vi "Create Channels.vi"(8 "error in (no error)":errorcluster) -> (0 "error out":errorcluster, 3 "Device Item Ref out":T3 format="%.0x")   [LabVIEW 2011, in "IVI DC Power Supply Custom Device.lvlib"]
uses:
  IVI DC Power Supply Custom Device.lvlib
  <vilib>/NI Veristand/Custom Device API/Custom Device Item Ref.ctl
  <vilib>/NI Veristand/Custom Device API/Custom Device Channel.ctl
  <vilib>/NI Veristand/Custom Device API/Custom Device Channel Type.ctl
  current behaviour.ctl
  Global.vi
  <vilib>/NI Veristand/Custom Device Tools/Custom Device Utility Library/NI VeriStand - Search for All Items by GUID.vi
  <vilib>/NI Veristand/Custom Device API/Set Item Property (U16).vi
  <vilib>/NI Veristand/Custom Device API/Get Item Property (U16).vi
  <vilib>/NI Veristand/Custom Device API/Custom Device API.lvlib
  <vilib>/NI Veristand/Custom Device Tools/Custom Device Utility Library/Custom Device Utility Library.lvlib
panel:
  in  "Output Channel":T1={"Type"=enum."Output", "Units"="", "Default Value"=0.0, "Faultable"=FALSE, "Scalable"=FALSE}
  in  "Input Channel":T1
  in  "Node Ptr":T3 format="%.0x"
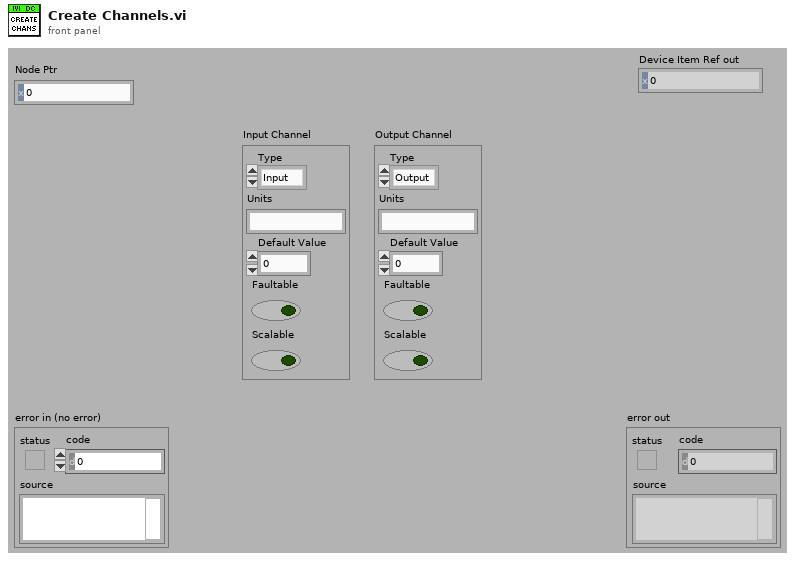
[diagram p1: front panel]
types:
  T1 = typedef "Custom Device API.lvlib/Custom Device Channel.ctl" = cluster{"Type":T2, "Units":string, "Default Value":dbl, "Faultable":bool, "Scalable":bool}
  T2 = typedef "Custom Device API.lvlib/Custom Device Channel Type.ctl" = enum16{"Input", "Output"}
  T3 = typedef "Custom Device API.lvlib/Custom Device Item Ref.ctl" = u64
  T4 = typedef "IVI DC Power Supply Custom Device.lvlib/current behaviour.ctl" = enum16{"Regulate", "Trip"}
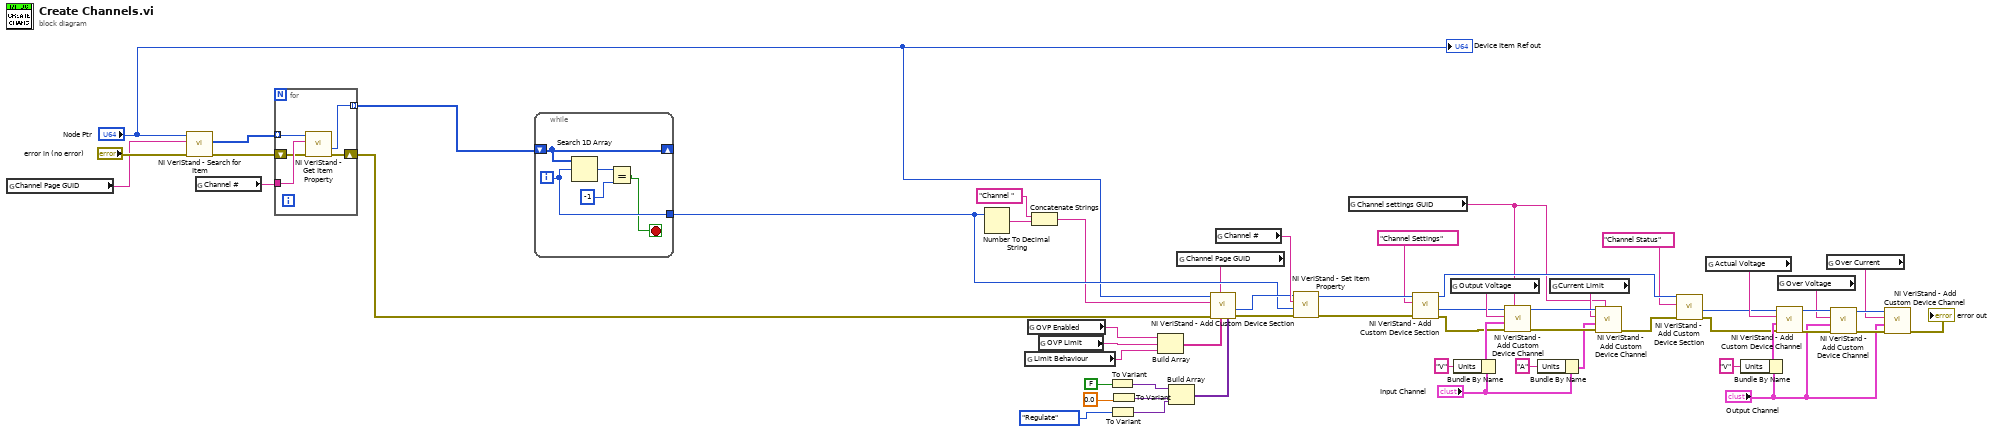
[diagram p0: block diagram]
diagram:
  n1 = global read "Global.vi" "Channel Page GUID"() -> (w1:string)
  n2 = call-poly <vilib>:"NI VeriStand - Search for Item.vi"("error in"="error in (no error)", "Item GUID"=w1, "Section Ref in"="Node Ptr") -> ("error out"=w2:errorcluster, "Item Refs"=w5:T3[])  [unwired: 5 in, 2 out]
  n3 = global read "Global.vi" "Channel #"() -> (w57:string)
  n4 = for {
    tunnel: w57 -> [w63]
    tunnel: w5 -> [w62] mode=indexing
    shift-right: [w60] -> w58
    shift-left: w2 -> [w61]
    tunnel: [w59] -> w6 mode=indexing
    n5 = call-poly <vilib>:"NI VeriStand - Get Item Property.vi"("error in (no error)"=w61, "Property Name"=w63, "Item Ref in"=w62) -> ("error out"=w60:errorcluster, "Value"=w59:u16)  [unwired: 5 in, 2 out]
  }
  n6 = while {
    shift-right: [w66] -> _
    shift-left: w6 -> [w66]
    tunnel: [w65] -> w46
    i -> [w65]
    stop <- w64 stop-if-true
    n7 = Search 1D Array(1D array=w66, element=w65) -> (index of element=w68:i32)  [unwired: 1 in]
    n8 = Equal?(x=w68, y=-1) -> (x = y?=w64:bool)
  }
  n9 = Number To Decimal String(number=w46) -> (decimal integer string=w49:string)  [unwired: 1 in]
  n10 = global read "Global.vi" "Limit Behaviour"() -> (w11:string)
  n11 = global read "Global.vi" "OVP Enabled"() -> (w56:string)
  n12 = Concatenate Strings("Channel " ("string"), w49) -> (w45:string)
  n13 = global read "Global.vi" "OVP Limit"() -> (w53:string)
  n14 = To Variant(anything=FALSE) -> (Variant=w55:variant)
  n15 = To Variant(anything=current_behaviour."Regulate" ("Enum")) -> (Variant=w9:variant)
  n16 = To Variant(anything=0.0) -> (Variant=w52:variant)
  n17 = Build Array(w56, w53, w11) -> (w39:string[])
  n18 = Build Array(w55, w52, w9) -> (w38:variant[])
  n19 = global read "Global.vi" "Channel Page GUID"() -> (w44:string)
  n20 = call <vilib>:"NI VeriStand - Add Custom Device Section.vi"("Property Values"=w38, "Property names"=w39, "GUID (Default Section)"=w44, "error in (no error)"=w58, "Section Name"=w45, "Parent Ref in"="Node Ptr") -> ("error out"=w51:errorcluster, "Section Ptr"=w47:T3)  [unwired: 2 in, 2 out]
  n21 = global read "Global.vi" "Channel #"() -> (w50:string)
  n22 = call-poly <vilib>:"NI VeriStand - Set Item Property.vi"("error in (no error)"=w51, "Value"=w46, "Property Name"=w50, "Item Ref in"=w47) -> ("error out"=w21:errorcluster, "Item Ref out"=w18:T3)  [unwired: 5 in, 1 out]
  n23 = global read "Global.vi" "Channel settings GUID"() -> (w7:string)
  n24 = call <vilib>:"NI VeriStand - Add Custom Device Section.vi"("error in (no error)"=w21, "Section Name"="Channel Settings", "Parent Ref in"=w18) -> ("error out"=w20:errorcluster, "Section Ptr"=w19:T3, "Parent Ref out"=w13:T3)  [unwired: 5 in, 1 out]
  n25 = global read "Global.vi" "Output Voltage"() -> (w42:string)
  n26 = Bundle By Name(cluster="Input Channel", "Units"="V") -> (w28:T1)
  n27 = call <vilib>:"NI VeriStand - Add Custom Device Channel.vi"("GUID (Default Channel)"=w7, "error in (no error)"=w20, "Channel"=w28, "Channel Name"=w42, "Parent Ref in"=w19) -> ("error out"=w40:errorcluster, "Parent Ref out"=w43:T3)  [unwired: 3 in, 2 out]
  n28 = Bundle By Name(cluster="Input Channel", "Units"="A") -> (w27:T1)
  n29 = global read "Global.vi" "Current Limit"() -> (w41:string)
  n30 = call <vilib>:"NI VeriStand - Add Custom Device Channel.vi"("GUID (Default Channel)"=w7, "error in (no error)"=w40, "Channel"=w27, "Channel Name"=w41, "Parent Ref in"=w43) -> ("error out"=w16:errorcluster)  [unwired: 3 in, 3 out]
  n31 = call <vilib>:"NI VeriStand - Add Custom Device Section.vi"("error in (no error)"=w16, "Section Name"="Channel Status", "Parent Ref in"=w13) -> ("error out"=w15:errorcluster, "Section Ptr"=w14:T3)  [unwired: 5 in, 2 out]
  n32 = global read "Global.vi" "Actual Voltage"() -> (w32:string)
  n33 = Bundle By Name(cluster="Output Channel", "Units"="V") -> (w22:T1)
  n34 = call <vilib>:"NI VeriStand - Add Custom Device Channel.vi"("error in (no error)"=w15, "Channel"=w22, "Channel Name"=w32, "Parent Ref in"=w14) -> ("error out"=w35:errorcluster, "Parent Ref out"=w34:T3)  [unwired: 4 in, 2 out]
  n35 = global read "Global.vi" "Over Voltage"() -> (w31:string)
  n36 = global read "Global.vi" "Over Current"() -> (w30:string)
  n37 = call <vilib>:"NI VeriStand - Add Custom Device Channel.vi"("error in (no error)"=w35, "Channel"="Output Channel", "Channel Name"=w31, "Parent Ref in"=w34) -> ("error out"=w36:errorcluster, "Parent Ref out"=w33:T3)  [unwired: 4 in, 2 out]
  n38 = call <vilib>:"NI VeriStand - Add Custom Device Channel.vi"("error in (no error)"=w36, "Channel"="Output Channel", "Channel Name"=w30, "Parent Ref in"=w33) -> ("error out"=→"error out":errorcluster)  [unwired: 4 in, 3 out]
  "Device Item Ref out" <- "Node Ptr"
